vi "Turn PID.vi"(11 "Setpoint":dbl) -> (3 "Done":bool)   [LabVIEW 2015]
uses:
  <vilib>/Rock Robotics/Network Tables/NT Read Number.vi
  <vilib>/Rock Robotics/WPI/Utilities/WPI_GetSetVariantRefNum.vi
  <vilib>/addons/control/pid/pid.llb/PID (DBL).vi
  <vilib>/addons/control/pid/NI_PID_pid.lvlib
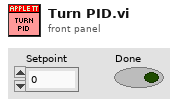
[diagram p1: front panel]
types:
  T1 = cluster{"proportional gain (Kc)":dbl, "integral time (Ti, min)":dbl, "derivative time (Td, min)":dbl}
  T2 = typedef "WPI_RobotDriveDevRef.ctl" = cluster{"DevStatus":errorcluster, "Motors[]":T3[], "Square Inputs":bool, "Max Output":dbl}
  T3 = typedef "WPI_MotorControlDeviceRef.ctl" = cluster{"DeviceStatus":errorcluster, "Type":T4, "PWM":cluster{"PWM Channel":T5, "DeadBand":T6}, "CAN":cluster{"Device Number":u8, "Control Mode":T7, "Semaphore":T8, "Max Vout":dbl, "TalonSRX Control Mode":T9}, "Invert":bool}
  T4 = typedef "WPI_MotorControlType.ctl" = enum16{"PWM", "CAN", "CANTalonSRX"}
  T5 = typedef "FPGA_DIOPWMChannel.ctl" = enum8{"PWM 0", "PWM 1", "PWM 2", "PWM 3", "PWM 4", "PWM 5", "PWM 6", "PWM 7", "PWM 8", "PWM 9", "PWM MXP 0", "PWM MXP 1", "PWM MXP 2", "PWM MXP 3", "PWM MXP 4", "PWM MXP 5", "PWM MXP 6", "PWM MXP 7", "PWM MXP 8", "PWM MXP 9", "Invalid"}
  T6 = typedef "WPI_PWMDeadband.ctl" = cluster{"Name":string, "maxPositivePwm":i32, "minPositivePwm":i32, "centerPwm":i32, "maxNegativePwm":i32, "minNegativePwm":i32, "angularRange":u16}
  T7 = typedef "WPI_CANJaguar_ControlMode.ctl" = enum8{"Percent VBus", "Current", "Speed", "Position", "Voltage"}
  T8 = typedef "Semaphore RefNum" = refnum<k1>
  T9 = typedef "WPI_CANTalonSRX_APIControlMode.ctl" = enum8{"Percent VBus", "Speed", "Position", "Slave", "Unchanged / Invalid", "Voltage Compensation", "Current", "Motion Profile"}
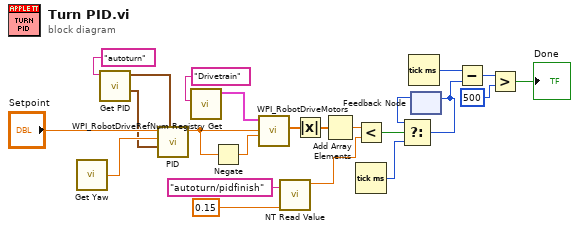
[diagram p0: block diagram]
diagram:
  n1 = call "Get Yaw.vi"() -> ("Angle"=w10:dbl)  [unwired: 1 in]
  n2 = call "Get PID.vi"("Subsystem"="autoturn") -> ("PID Gains"=w8:T1, "output range"=w7:cluster{"output high":dbl, "output low":dbl})  [unwired: 8 in]
  n3 = call-poly <vilib>:"PID.vi"("output range"=w7, "PID gains"=w8, "process variable"=w10, "setpoint"="Setpoint") -> ("output"=w11:dbl)  [unwired: 6 in, 1 out]
  n4 = call <vilib>:"WPI_RobotDriveRefNum Registry Get.vi"("refnum name"="Drivetrain") -> ("RobotDriveDevRef"=w4:T2)  [unwired: 9 in, 1 out]
  n5 = Negate(x=w11) -> (-x=w12:dbl)
  n6 = call <vilib>:"WPI_RobotDriveMotors.vi"("RightSpeed"=w12, "LeftSpeed"=w11, "RobotDriveDevRef"=w4) -> ("Motor Values"=w22:dbl[])  [unwired: 6 in, 2 out]
  n7 = call-poly <vilib>:"NT Read Value.vi"("Default Value"=0.15, "Name"="autoturn/pidfinish") -> ("Numeric"=w1:dbl)  [unwired: 8 in, 1 out]
  n8 = Absolute Value(x=w22) -> (abs(x)=w13:dbl[])
  n9 = Add Array Elements(numeric array=w13) -> (sum=w14:dbl)
  n10 = Less?(x=w14, y=w1) -> (x < y?=w15:bool)
  n11 = Tick Count (ms)() -> (millisecond timer value=w16:u32)
  n12 = Tick Count (ms)() -> (millisecond timer value=w18:u32)
  n13 = feedback #1() -> (w17:u32)  [unwired: 1 in]
  n14 = Select(t=w17, s=w15, f=w16) -> (s? t:f=w19:u32)
  n15 = feedback-in #1(w19) -> ()
  n16 = Subtract(x=w18, y=w19) -> (x-y=w20:u32)
  n17 = Greater?(x=w20, y=u32 500) -> (0:→"Done":bool)
